vi "CalculateRMS.vi"(8 "error in (no error)":errorcluster, 11 "Waveform":waveform(dbl)) -> (0 "error out":errorcluster, 3 "RMS value":dbl)   [LabVIEW 2016, in "McsaAnalysisFunctions.lvlib"]
uses:
  <vilib>/addons/InsightCM/Utilities/Analysis/MCSA/McsaAnalysisFunctions.lvlib
  <vilib>/addons/Electrical Power/Basic/Measurement/RMS (1 Channel).vi
  <vilib>/addons/Electrical Power/Basic/NI_EP_Basic.lvlib
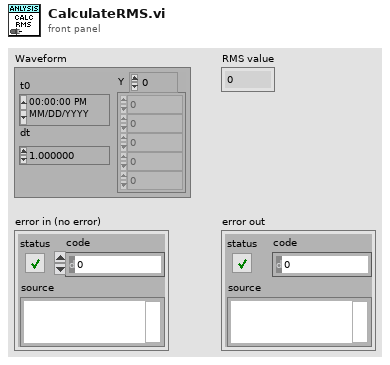
[diagram p1: front panel]
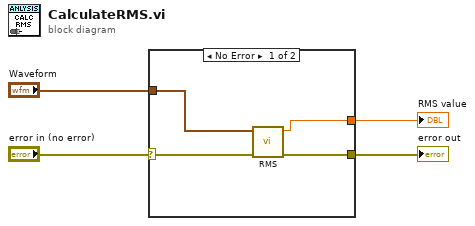
[diagram p0: block diagram]
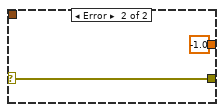
[diagram p2: hidden frame]
diagram:
  n1 = case shown="No Error" "error in (no error)" {
    selector: "error in (no error)" -> [w8 w10]
    tunnel: [w6 -1.0 ("RMS value")] -> w4
    tunnel: [w7 w10] -> w3
    tunnel: "Waveform" -> [w5 _]
    frame No Error {
      n2 = call-poly <vilib>:"RMS.vi"("error in (no error)"=w8, "waveform"=w5) -> ("error out"=w7:errorcluster, "RMS value"=w6:dbl)  [unwired: 8 in]
    }
    frame Error {
    }
  }
  "RMS value" <- w4
  "error out" <- w3
